vi "Open New  WorkBook.vi"(2 "error in (no error)":errorcluster, 4 "Excel._Application":refnum<k7>) -> (0 "error out":errorcluster, 1 "Excel._Workbook":refnum<k7>)   [LabVIEW 2012]
doc: "Opens a WorkBook by name. Takes a Application Refnum as input. If the name is not connected or its string length is zero then it opens a new Workbook else it adds the specified workBook to the WorkBooks object collection."
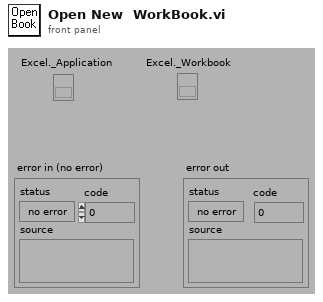
[diagram p1: front panel]
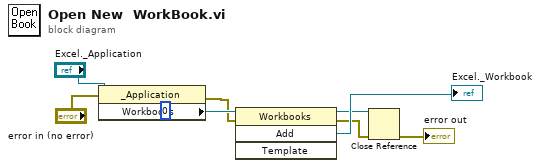
[diagram p0: block diagram]
diagram:
  (unwired) 0
  n1 = property class="_Application"(reference="Excel._Application", error in="error in (no error)") -> (error out=w5:errorcluster, "Workbooks"=w6:refnum<k7>)  [unwired: 1 out]
  n2 = invoke class="Workbooks" method="Add"(reference=w6, error in=w5) -> (reference out=w1:refnum<k7>, error out=w3:errorcluster, "Add"=→"Excel._Workbook":refnum<k7>)  [unwired: 2 in, 1 out]
  n3 = Close Reference(reference=w1, error in (no error)=w3) -> (error out=→"error out":errorcluster)
